vi "XY_MoveToPosition_RT.vi"(9 "ReturnDataStatus":T1, 10 "Positon (X / Y)":i32[](array[numeric])) -> (2 "Command":string)   [LabVIEW 2017]
uses:
  sobot structures/ReturnDataStatus.ctl
  sobot structures/SoBot_CommandTypes.ctl
  sobot structures/XY_Commands.ctl
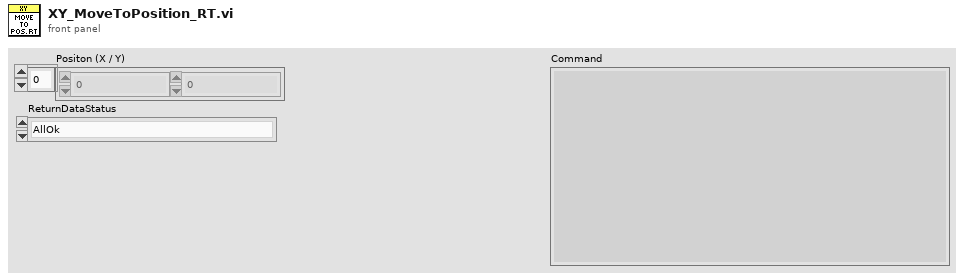
[diagram p1: front panel]
types:
  T1 = typedef "ReturnDataStatus.ctl" = enum16{"AllOk", "Error"}
  T2 = typedef "XY_Commands.ctl" = enum16{"XY_Initialize", "XY_MoveToPosition", "XY_MarkTarget", "XY_LockMotors", "XY_UnlockMotors"}
  T3 = typedef "SoBot_CommandTypes.ctl" = enum16{"General_Command", "XY_Command", "Z_Command", "Plattform_Command"}
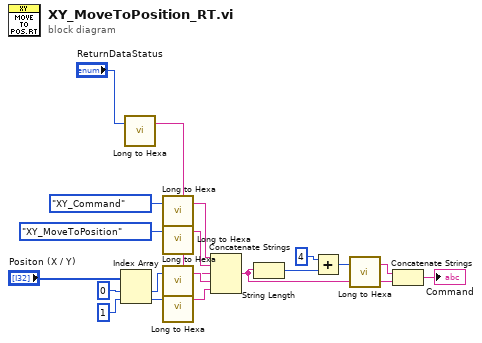
[diagram p0: block diagram]
diagram:
  n1 = Index Array(array="Positon (X / Y)", index #1=0 ("index"), index #2=1 ("index")) -> (element #1=w8:i32, element #2=w7:i32)
  n2 = call "Long to Hexa.vi"("Long"="ReturnDataStatus") -> ("Hexa"=w2:string)  [unwired: 2 in]
  n3 = call "Long to Hexa.vi"("Long"=SoBot_CommandTypes."XY_Command" ("SoBot_CommandTypes")) -> ("Hexa"=w19:string)  [unwired: 2 in]
  n4 = call "Long to Hexa.vi"("Long"=XY_Commands."XY_MoveToPosition" ("XY_Command")) -> ("Hexa"=w18:string)  [unwired: 2 in]
  n5 = call "Long to Hexa.vi"("Long"=w8) -> ("Hexa"=w3:string)  [unwired: 2 in]
  n6 = call "Long to Hexa.vi"("Long"=w7) -> ("Hexa"=w4:string)  [unwired: 2 in]
  n7 = Concatenate Strings(w19, w18, w2, w3, w4) -> (w13:string)
  n8 = String Length(string=w13) -> (length=w17:i32)
  n9 = Add(x=4, y=w17) -> (x+y=w15:i32)
  n10 = call "Long to Hexa.vi"("Long"=w15) -> ("Hexa"=w14:string)  [unwired: 2 in]
  n11 = Concatenate Strings(w14, w13) -> (→"Command":string)
